vi "Lab Panel V4.87.vi"() -> ()   [LabVIEW 2013] (continued)
                n1786 = property on="JIG TEST" class="Clust (strict)"() -> ("DisabledEnum"=w3336:T16)  [unwired: 2 in, 2 out]
                n1787 = Equal?(x=w3336, y=2) -> (x = y?=w3335:bool)
                n1788 = Equal?(x=w3339, y=0) -> (x = y?=w3337:bool)
                n1789 = And(x=w3337, y=w3335) -> (x .and. y?=w3334:bool)
                n1790 = case shown="True" w3334 {
                  frame False {
                  }
                  frame True {
                    n1791 = local read "run lab01-1"() -> (w3350:bool)
                    n1792 = local read "run lab01-2"() -> (w3349:bool)
                    n1793 = local read "run lab02-1"() -> (w3348:bool)
                    n1794 = local read "run lab02-2"() -> (w3347:bool)
                    n1795 = local read "run lab03-1"() -> (w3346:bool)
                    n1796 = local read "run lab03-2"() -> (w3345:bool)
                    n1797 = local read "run lab04-1"() -> (w3344:bool)
                    n1798 = local read "run lab04-2"() -> (w3343:bool)
                    n1799 = local read "run lab05-1"() -> (w3342:bool)
                    n1800 = local read "run lab05-2"() -> (w3341:bool)
                    n1801 = local write "JIG LAB03-2"(w3345) -> ()
                    n1802 = local write "JIG LAB01-1"(w3350) -> ()
                    n1803 = local write "JIG LAB01-2"(w3349) -> ()
                    n1804 = local write "JIG LAB02-1"(w3348) -> ()
                    n1805 = local write "JIG LAB02-2"(w3347) -> ()
                    n1806 = local write "JIG LAB03-1"(w3346) -> ()
                    n1807 = local write "JIG LAB04-1"(w3344) -> ()
                    n1808 = local write "JIG LAB04-2"(w3343) -> ()
                    n1809 = local write "JIG LAB05-1"(w3342) -> ()
                    n1810 = local write "JIG LAB05-2"(w3341) -> ()
                  }
                }
              }
              frame #1 {
                # "jig off"
                n1811 = local read "jig cycle"() -> (w3357:dbl)
                n1812 = local read "on loops"() -> (w3356:dbl)
                n1813 = property on="JIG TEST" class="Clust (strict)"() -> ("DisabledEnum"=w3355:T16)  [unwired: 2 in, 2 out]
                n1814 = Equal?(x=w3355, y=2) -> (x = y?=w3353:bool)
                n1815 = Equal?(x=w3357, y=w3356) -> (x = y?=w3352:bool)
                n1816 = And(x=w3352, y=w3353) -> (x .and. y?=w3351:bool)
                n1817 = case shown="True" w3351 {
                  frame False {
                  }
                  frame True {
                    w3408 = FALSE
                    w3409 = TRUE
                    w3407 = 2
                    n1818 = local read "SELECT LAB05-2"() -> (w3398:T3)
                    n1819 = local read "SELECT LAB04-2"() -> (w3400:T3)
                    n1820 = local read "SELECT LAB04-1"() -> (w3401:T3)
                    n1821 = local read "SELECT LAB05-1"() -> (w3399:T3)
                    n1822 = local read "SELECT LAB03-2"() -> (w3402:T3)
                    n1823 = local read "SELECT LAB02-1"() -> (w3405:T3)
                    n1824 = local read "SELECT LAB03-1"() -> (w3403:T3)
                    n1825 = local read "SELECT LAB02-2"() -> (w3404:T3)
                    n1826 = local read "SELECT LAB01-2"() -> (w3406:T3)
                    n1827 = local read "run lab05-1"() -> (w3368:bool)
                    n1828 = local read "run lab05-2"() -> (w3367:bool)
                    n1829 = local read "SELECT LAB01-1"() -> (w3410:T3)
                    n1830 = local read "run lab04-2"() -> (w3369:bool)
                    n1831 = local read "run lab04-1"() -> (w3370:bool)
                    n1832 = local read "run lab01-1"() -> (w3386:bool)
                    n1833 = local read "run lab01-2"() -> (w3375:bool)
                    n1834 = local read "run lab03-2"() -> (w3371:bool)
                    n1835 = local read "run lab03-1"() -> (w3372:bool)
                    n1836 = local read "run lab02-1"() -> (w3374:bool)
                    n1837 = local read "run lab02-2"() -> (w3373:bool)
                    n1838 = Equal?(x=w3407, y=w3403) -> (x = y?=w3381:bool)
                    n1839 = Equal?(x=w3407, y=w3402) -> (x = y?=w3380:bool)
                    n1840 = Equal?(x=w3407, y=w3401) -> (x = y?=w3379:bool)
                    n1841 = Equal?(x=w3407, y=w3400) -> (x = y?=w3378:bool)
                    n1842 = Equal?(x=w3407, y=w3399) -> (x = y?=w3377:bool)
                    n1843 = Equal?(x=w3407, y=w3398) -> (x = y?=w3376:bool)
                    n1844 = Equal?(x=w3407, y=w3410) -> (x = y?=w3387:bool)
                    n1845 = Equal?(x=w3407, y=w3405) -> (x = y?=w3383:bool)
                    n1846 = Equal?(x=w3407, y=w3404) -> (x = y?=w3382:bool)
                    n1847 = Equal?(x=w3407, y=w3406) -> (x = y?=w3384:bool)
                    n1848 = And(x=w3378, y=w3369) -> (x .and. y?=w3360:bool)
                    n1849 = And(x=w3381, y=w3372) -> (x .and. y?=w3363:bool)
                    n1850 = And(x=w3379, y=w3370) -> (x .and. y?=w3361:bool)
                    n1851 = And(x=w3376, y=w3367) -> (x .and. y?=w3358:bool)
                    n1852 = And(x=w3382, y=w3373) -> (x .and. y?=w3364:bool)
                    n1853 = And(x=w3380, y=w3371) -> (x .and. y?=w3362:bool)
                    n1854 = And(x=w3377, y=w3368) -> (x .and. y?=w3359:bool)
                    n1855 = And(x=w3384, y=w3375) -> (x .and. y?=w3366:bool)
                    n1856 = And(x=w3387, y=w3386) -> (x .and. y?=w3385:bool)
                    n1857 = And(x=w3383, y=w3374) -> (x .and. y?=w3365:bool)
                    n1858 = Select(t=w3409, s=w3385, f=w3408) -> (s? t:f=w3388:bool)
                    n1859 = Select(t=w3409, s=w3366, f=w3408) -> (s? t:f=w3389:bool)
                    n1860 = Select(t=w3409, s=w3365, f=w3408) -> (s? t:f=w3390:bool)
                    n1861 = Select(t=w3409, s=w3364, f=w3408) -> (s? t:f=w3391:bool)
                    n1862 = Select(t=w3409, s=w3363, f=w3408) -> (s? t:f=w3392:bool)
                    n1863 = Select(t=w3409, s=w3362, f=w3408) -> (s? t:f=w3393:bool)
                    n1864 = Select(t=w3409, s=w3361, f=w3408) -> (s? t:f=w3394:bool)
                    n1865 = Select(t=w3409, s=w3360, f=w3408) -> (s? t:f=w3395:bool)
                    n1866 = Select(t=w3409, s=w3359, f=w3408) -> (s? t:f=w3396:bool)
                    n1867 = Select(t=w3409, s=w3358, f=w3408) -> (s? t:f=w3397:bool)
                    n1868 = local write "JIG LAB03-2"(w3393) -> ()
                    n1869 = local write "JIG LAB02-1"(w3390) -> ()
                    n1870 = local write "JIG LAB02-2"(w3391) -> ()
                    n1871 = local write "JIG LAB01-2"(w3389) -> ()
                    n1872 = local write "JIG LAB03-1"(w3392) -> ()
                    n1873 = local write "JIG LAB01-1"(w3388) -> ()
                    n1874 = local write "JIG LAB05-2"(w3397) -> ()
                    n1875 = local write "JIG LAB04-1"(w3394) -> ()
                    n1876 = local write "JIG LAB05-1"(w3396) -> ()
                    n1877 = local write "JIG LAB04-2"(w3395) -> ()
                  }
                }
              }
            }
          }
          frame #9 {
            # "enable  jig test output if no test busy"
            n1878 = property on="JIG TEST" class="Clust (strict)"() -> ("DisabledEnum"=w3413:T16)  [unwired: 2 in, 2 out]
            n1879 = Equal?(x=w3413, y=0) -> (x = y?=w3411:bool)
            n1880 = case shown="True" w3411 {
              frame False {
              }
              frame True {
                n1881 = local read "JIG TEST"() -> (w3424:T10)
                n1882 = Unbundle(w3424) -> ("LAB01-1"=w3423:bool, "LAB01-2"=w3422:bool, "LAB02-1"=w3421:bool, "LAB02-2"=w3420:bool, "LAB03-1"=w3419:bool, "LAB03-2"=w3418:bool, "LAB04-1"=w3417:bool, "LAB04-2"=w3416:bool, "LAB05-1"=w3415:bool, "LAB05-2"=w3414:bool)
                n1883 = local write "JIG LAB05-1"(w3415) -> ()
                n1884 = local write "JIG LAB05-2"(w3414) -> ()
                n1885 = local write "JIG LAB04-1"(w3417) -> ()
                n1886 = local write "JIG LAB04-2"(w3416) -> ()
                n1887 = local write "JIG LAB03-2"(w3418) -> ()
                n1888 = local write "JIG LAB01-1"(w3423) -> ()
                n1889 = local write "JIG LAB02-1"(w3421) -> ()
                n1890 = local write "JIG LAB03-1"(w3419) -> ()
                n1891 = local write "JIG LAB01-2"(w3422) -> ()
                n1892 = local write "JIG LAB02-2"(w3420) -> ()
              }
            }
          }
          frame #10 {
            # "drive digital output"
            n1893 = local read "O/I  LAB05-2"() -> (w3431:bool)
            n1894 = local read "O/I  LAB05-1"() -> (w3433:bool)
            n1895 = local read "JIG LAB05-2"() -> (w3430:bool)
            n1896 = local read "O/I  LAB04-2"() -> (w3435:bool)
            n1897 = local read "JIG LAB05-1"() -> (w3432:bool)
            n1898 = local read "JIG LAB04-2"() -> (w3434:bool)
            n1899 = local read "O/I  LAB03-1"() -> (w3440:bool)
            n1900 = local read "O/I  LAB04-1"() -> (w3436:bool)
            n1901 = local read "O/I  LAB02-1"() -> (w3444:bool)
            n1902 = local read "O/I  LAB02-2"() -> (w3442:bool)
            n1903 = local read "O/I  LAB03-2"() -> (w3438:bool)
            n1904 = local read "JIG LAB04-1"() -> (w3429:bool)
            n1905 = local read "JIG LAB03-2"() -> (w3437:bool)
            n1906 = local read "O/I  LAB01-2"() -> (w3446:bool)
            n1907 = local read "JIG LAB02-1"() -> (w3443:bool)
            n1908 = local read "JIG LAB02-2"() -> (w3441:bool)
            n1909 = local read "JIG LAB03-1"() -> (w3439:bool)
            n1910 = local read "O/I  LAB01-1"() -> (w3448:bool)
            n1911 = local read "JIG LAB01-2"() -> (w3445:bool)
            n1912 = local read "JIG LAB01-1"() -> (w3447:bool)
            n1913 = Build Array(w3435, w3434, w3433, w3432, w3431, w3430) -> (w3426:bool[])
            n1914 = Build Array(w3441, w3440, w3439, w3438, w3437, w3436, w3429) -> (w3427:bool[])
            n1915 = Build Array(w3448, w3447, w3446, w3445, w3444, w3443, w3442) -> (w3428:bool[])
            n1916 = local read "simulate"() -> (w3425:bool)
            n1917 = case shown="False" w3425 {
              tunnel: w3428 -> [w3451 _]
              tunnel: w3427 -> [w3450 _]
              tunnel: w3426 -> [w3449 _]
              frame False {
                n1918 = call "sub vi - Drive Relays All v6.vi"("Array #2"=w3449, "Array #1"=w3450, "Array #0"=w3451) -> ()  [unwired: 8 in, 1 out]
              }
              frame True {
              }
            }
          }
          frame #11 {
            # "get analog values"
            n1919 = local read "on loops"() -> (w3458:dbl)
            n1920 = local read "jig cycle"() -> (w3455:dbl)
            n1921 = Add(x=w3458, y=1) -> (x+y=w3456:dbl)
            n1922 = Equal?(x=w3455, y=1) -> (x = y?=w3452:bool)
            n1923 = Equal?(x=w3455, y=w3456) -> (x = y?=w3454:bool)
            n1924 = Or(x=w3452, y=w3454) -> (x .or. y?=w3453:bool)
            n1925 = global write "Global display 3.vi" "cycle O/F"(w3452) -> ()
            n1926 = case shown="True" w3453 {
              tunnel: w3452 -> [_ w3460]
              frame False {
              }
              frame True {
                n1927 = local read "simulate"() -> (w3463:bool)
                n1928 = case shown="True" w3463 {
                  tunnel: [w3472 errorcluster[] [] ("array ERROR")] -> w3471
                  tunnel: [w3479 0.3 ("Analog loop time")] -> w3470
                  tunnel: [w3478 dynamicdata[] [] ("array GRAPH")] -> w3469
                  tunnel: [w3477 w3480] -> w3468
                  tunnel: [w3476 w3480] -> w3467
                  tunnel: [w3475 w3480] -> w3466
                  tunnel: [w3474 w3480] -> w3465
                  tunnel: [w3473 w3480] -> w3464
                  tunnel: w3460 -> [_ w3486]
                  frame False {
                    n1929 = call "sub vi - Read Analog All v8.11.vi"() -> ("Analog loop time"=w3479:dbl, "array GRAPH"=w3478:dynamicdata[], "LAB01"=w3477:T26, "LAB02"=w3476:T27, "LAB03"=w3475:T28, "LAB04"=w3474:T29, "array ERROR"=w3472:errorcluster[], "LAB05"=w3473:T30)  [unwired: 8 in]
                  }
                  frame True {
                    n1930 = local read "ON amps"() -> (w3485:dbl)
                    n1931 = local read "OFF amps"() -> (w3484:dbl)
                    n1932 = local read "VOLTS"() -> (w3482:dbl)
                    n1933 = local read "PF"() -> (w3481:dbl)
                    n1934 = Select(t=w3485, s=w3486, f=w3484) -> (s? t:f=w3483:dbl)
                    n1935 = Bundle("OFF amps"=w3483, "VOLTS"=w3482, "PF"=w3481, "OFF amps"=w3483, "VOLTS"=w3482, "PF"=w3481) -> (w3480:T31)  [unwired: 1 in]
                  }
                }
                n1936 = local read "simulate"() -> (w3462:bool)
                n1937 = stacked-sequence {
                  tunnel: w3471 -> [w3494 _ _ _ _ _]
                  tunnel: w3470 -> [w3493 _ _ _ _ _]
                  tunnel: w3469 -> [w3490 _ _ _ _ _]
                  tunnel: w3468 -> [_ w3541 _ _ _ _]
                  tunnel: w3467 -> [_ _ w3548 _ _ _]
                  tunnel: w3466 -> [_ _ _ w3577 _ _]
                  tunnel: w3465 -> [_ _ _ _ w3604 _]
                  tunnel: w3464 -> [_ _ _ _ _ w3633]
                  tunnel: w3462 -> [_ w3519 w3547 w3575 w3603 w3631]
                  tunnel: T14 {"1  (A) cal"=1.0, "1 (V) cal"=1.0, "1 (PF) cal"=1.0, "1 (TL) cal"=1.0, "1 (TN) cal"=1.0, "2 (A) cal"=1.0, "2 (V) cal"=1.0, "2 (PF) cal"=1.0, "2 (TL) cal"=1.0, "2 (TN) cal"=1.0} ("CAL LAB01") -> [_ w3518 w3546 w3574 w3602 w3630]
                  frame #0 {
                    n1938 = local write "AI"(TRUE) -> ()
                    n1939 = global write "Global 1.vi" "RATE(Hz)"("RATE (Hz)") -> ()
                    n1940 = global write "Global 1.vi" "SAMPLES"("SAMPLES") -> ()
                    n1941 = Index Array(array=w3490, index=6) -> (element=→"LAB04-1 (GRAPH)":dynamicdata)
                    n1942 = Index Array(array=w3490, index=7) -> (element=→"LAB04-2 (GRAPH)":dynamicdata)
                    n1943 = Index Array(array=w3490, index=9) -> (element=→"LAB05-2 (GRAPH)":dynamicdata)
                    n1944 = Index Array(array=w3490, index=8) -> (element=→"LAB05-1 (GRAPH)":dynamicdata)
                    n1945 = Index Array(array=w3490, index=5) -> (element=→"LAB03-2 (GRAPH)":dynamicdata)
                    n1946 = Index Array(array=w3490, index=0) -> (element=→"LAB01-1 (GRAPH)":dynamicdata)
                    n1947 = Index Array(array=w3490, index=1) -> (element=→"LAB01-2 (GRAPH)":dynamicdata)
                    n1948 = Index Array(array=w3490, index=2) -> (element=→"LAB02-1 (GRAPH)":dynamicdata)
                    n1949 = Index Array(array=w3490, index=3) -> (element=→"LAB02-2 (GRAPH)":dynamicdata)
                    n1950 = Index Array(array=w3490, index=4) -> (element=→"LAB03-1 (GRAPH)":dynamicdata)
                    "AI loop time" <- w3493
                    "Analog Error Array" <- w3494
                  }
                  frame #1 {
                    n1951 = case shown="False" w3519 {
                      tunnel: [w3542 w3543] -> w3540
                      tunnel: w3518 -> [_ w3543]
                      frame False {
                        n1952 = local read "CAL LAB01"() -> (w3542:T14)
                      }
                      frame True {
                      }
                    }
                    n1953 = Unbundle By Name(w3541) -> ("OFF amps"=w3539:dbl, "VOLTS"=w3538:dbl, "PF"=w3537:dbl, "OFF amps"=w3536:dbl, "VOLTS"=w3535:dbl, "PF"=w3534:dbl)
                    n1954 = Unbundle By Name(w3540) -> ("1  (A) cal"=w3533:dbl, "1 (V) cal"=w3532:dbl, "1 (PF) cal"=w3531:dbl, "2 (A) cal"=w3530:dbl, "2 (V) cal"=w3529:dbl, "2 (PF) cal"=w3528:dbl)  [unwired: 4 out]
                    n1955 = Multiply(x=w3539, y=w3533) -> (x*y=w3526:dbl)
                    n1956 = Multiply(x=w3538, y=w3532) -> (x*y=w3525:dbl)
                    n1957 = Multiply(x=w3537, y=w3531) -> (x*y=w3524:dbl)
                    n1958 = Multiply(x=w3536, y=w3530) -> (x*y=w3522:dbl)
                    n1959 = Multiply(x=w3535, y=w3529) -> (x*y=w3521:dbl)
                    n1960 = Multiply(x=w3534, y=w3528) -> (x*y=w3520:dbl)
                    n1961 = local read "SIG LAB01-1"() -> (w3527:T2)
                    n1962 = local read "SIG LAB01-2"() -> (w3523:T2)
                    n1963 = Bundle By Name(cluster=w3527, "AMPS"=w3526, "VOLTS"=w3525, "PF"=w3524) -> (w3517:T2)
                    n1964 = Bundle By Name(cluster=w3523, "AMPS"=w3522, "VOLTS"=w3521, "PF"=w3520) -> (w3516:T2)
                    n1965 = global write "Global display 1.vi" "SIG LAB01-2"(w3516) -> ()
                    n1966 = global write "Global display 1.vi" "SIG LAB01-1"(w3517) -> ()
                    n1967 = local write "SIG LAB01-2"(w3516) -> ()
                    n1968 = local write "SIG LAB01-1"(w3517) -> ()
                  }
                  frame #2 {
                    n1969 = Unbundle By Name(w3548) -> ("OFF amps"=w3568:dbl, "VOLTS"=w3567:dbl, "PF"=w3566:dbl, "OFF amps"=w3565:dbl, "VOLTS"=w3564:dbl, "PF"=w3563:dbl)
                    n1970 = case shown="True" w3547 {
                      tunnel: [w3570 w3571] -> w3569
                      tunnel: w3546 -> [_ w3571]
                      frame False {
                        n1971 = local read "CAL LAB02"() -> (w3570:T15)
                      }
                      frame True {
                      }
                    }
                    n1972 = Unbundle By Name(w3569) -> ("1  (A) cal"=w3562:dbl, "1 (V) cal"=w3561:dbl, "1 (PF) cal"=w3560:dbl, "2 (A) cal"=w3559:dbl, "2 (V) cal"=w3558:dbl, "2 (PF) cal"=w3557:dbl)  [unwired: 4 out]
                    n1973 = Multiply(x=w3568, y=w3562) -> (x*y=w3555:dbl)
                    n1974 = Multiply(x=w3567, y=w3561) -> (x*y=w3554:dbl)
                    n1975 = Multiply(x=w3566, y=w3560) -> (x*y=w3553:dbl)
                    n1976 = Multiply(x=w3565, y=w3559) -> (x*y=w3551:dbl)
                    n1977 = Multiply(x=w3564, y=w3558) -> (x*y=w3550:dbl)
                    n1978 = Multiply(x=w3563, y=w3557) -> (x*y=w3549:dbl)
                    n1979 = local read "SIG LAB02-1"() -> (w3556:T2)
                    n1980 = local read "SIG LAB02-2"() -> (w3552:T2)
                    n1981 = Bundle By Name(cluster=w3556, "AMPS"=w3555, "VOLTS"=w3554, "PF"=w3553) -> (w3545:T2)
                    n1982 = Bundle By Name(cluster=w3552, "AMPS"=w3551, "VOLTS"=w3550, "PF"=w3549) -> (w3544:T2)
                    n1983 = global write "Global display 1.vi" "SIG LAB02-1"(w3545) -> ()
                    n1984 = local write "SIG LAB02-2"(w3544) -> ()
                    n1985 = global write "Global display 1.vi" "SIG LAB02-2"(w3544) -> ()
                    n1986 = local write "SIG LAB02-1"(w3545) -> ()
                  }
                  frame #3 {
                    n1987 = Unbundle By Name(w3577) -> ("OFF amps"=w3596:dbl, "VOLTS"=w3595:dbl, "PF"=w3594:dbl, "OFF amps"=w3593:dbl, "VOLTS"=w3592:dbl, "PF"=w3591:dbl)
                    n1988 = case shown="True" w3575 {
                      tunnel: [w3598 w3599] -> w3597
                      tunnel: w3574 -> [_ w3599]
                      frame False {
                        n1989 = local read "CAL LAB03"() -> (w3598:T14)
                      }
                      frame True {
                      }
                    }
                    n1990 = Unbundle By Name(w3597) -> ("1  (A) cal"=w3590:dbl, "1 (V) cal"=w3589:dbl, "1 (PF) cal"=w3588:dbl, "2 (A) cal"=w3587:dbl, "2 (V) cal"=w3586:dbl, "2 (PF) cal"=w3585:dbl)  [unwired: 4 out]
                    n1991 = Multiply(x=w3596, y=w3590) -> (x*y=w3583:dbl)
                    n1992 = Multiply(x=w3595, y=w3589) -> (x*y=w3576:dbl)
                    n1993 = Multiply(x=w3594, y=w3588) -> (x*y=w3582:dbl)
                    n1994 = Multiply(x=w3593, y=w3587) -> (x*y=w3580:dbl)
                    n1995 = Multiply(x=w3592, y=w3586) -> (x*y=w3579:dbl)
                    n1996 = Multiply(x=w3591, y=w3585) -> (x*y=w3578:dbl)
                    n1997 = local read "SIG LAB03-1"() -> (w3584:T2)
                    n1998 = local read "SIG LAB03-2"() -> (w3581:T2)
                    n1999 = Bundle By Name(cluster=w3584, "AMPS"=w3583, "VOLTS"=w3576, "PF"=w3582) -> (w3573:T2)
                    n2000 = Bundle By Name(cluster=w3581, "AMPS"=w3580, "VOLTS"=w3579, "PF"=w3578) -> (w3572:T2)
                    n2001 = global write "Global display 1.vi" "SIG LAB03-1"(w3573) -> ()
                    n2002 = global write "Global display 1.vi" "SIG LAB03-2"(w3572) -> ()
                    n2003 = local write "SIG LAB03-2"(w3572) -> ()
                    n2004 = local write "SIG LAB03-1"(w3573) -> ()
                  }
                  frame #4 {
                    n2005 = Unbundle By Name(w3604) -> ("OFF amps"=w3624:dbl, "VOLTS"=w3623:dbl, "PF"=w3622:dbl, "OFF amps"=w3621:dbl, "VOLTS"=w3620:dbl, "PF"=w3619:dbl)
                    n2006 = case shown="False" w3603 {
                      tunnel: [w3626 w3627] -> w3625
                      tunnel: w3602 -> [_ w3627]
                      frame False {
                        n2007 = local read "CAL LAB04"() -> (w3626:T14)
                      }
                      frame True {
                      }
                    }
                    n2008 = Unbundle By Name(w3625) -> ("1  (A) cal"=w3618:dbl, "1 (V) cal"=w3617:dbl, "1 (PF) cal"=w3616:dbl, "2 (A) cal"=w3615:dbl, "2 (V) cal"=w3614:dbl, "2 (PF) cal"=w3613:dbl)  [unwired: 4 out]
                    n2009 = Multiply(x=w3624, y=w3618) -> (x*y=w3611:dbl)
                    n2010 = Multiply(x=w3623, y=w3617) -> (x*y=w3610:dbl)
                    n2011 = Multiply(x=w3622, y=w3616) -> (x*y=w3609:dbl)
                    n2012 = Multiply(x=w3621, y=w3615) -> (x*y=w3607:dbl)
                    n2013 = Multiply(x=w3620, y=w3614) -> (x*y=w3606:dbl)
                    n2014 = Multiply(x=w3619, y=w3613) -> (x*y=w3605:dbl)
                    n2015 = local read "SIG LAB04-1"() -> (w3612:T2)
                    n2016 = local read "SIG LAB04-2"() -> (w3608:T2)
                    n2017 = Bundle By Name(cluster=w3612, "AMPS"=w3611, "VOLTS"=w3610, "PF"=w3609) -> (w3601:T2)
                    n2018 = Bundle By Name(cluster=w3608, "AMPS"=w3607, "VOLTS"=w3606, "PF"=w3605) -> (w3600:T2)
                    n2019 = global write "Global display 1.vi" "SIG LAB04-2"(w3600) -> ()
                    n2020 = global write "Global display 1.vi" "SIG LAB04-1"(w3601) -> ()
                    n2021 = local write "SIG LAB04-2"(w3600) -> ()
                    n2022 = local write "SIG LAB04-1"(w3601) -> ()
                  }
                  frame #5 {
                    n2023 = Unbundle By Name(w3633) -> ("OFF amps"=w3652:dbl, "VOLTS"=w3632:dbl, "PF"=w3651:dbl, "OFF amps"=w3650:dbl, "VOLTS"=w3649:dbl, "PF"=w3648:dbl)
                    n2024 = case shown="False" w3631 {
                      tunnel: [w3654 w3655] -> w3653
                      tunnel: w3630 -> [_ w3655]
                      frame False {
                        n2025 = local read "CAL LAB05"() -> (w3654:T14)
                      }
                      frame True {
                      }
                    }
                    n2026 = Unbundle By Name(w3653) -> ("1  (A) cal"=w3647:dbl, "1 (V) cal"=w3646:dbl, "1 (PF) cal"=w3645:dbl, "2 (A) cal"=w3644:dbl, "2 (V) cal"=w3643:dbl, "2 (PF) cal"=w3642:dbl)  [unwired: 4 out]
                    n2027 = Multiply(x=w3652, y=w3647) -> (x*y=w3640:dbl)
                    n2028 = Multiply(x=w3632, y=w3646) -> (x*y=w3639:dbl)
                    n2029 = Multiply(x=w3651, y=w3645) -> (x*y=w3638:dbl)
                    n2030 = Multiply(x=w3650, y=w3644) -> (x*y=w3636:dbl)
                    n2031 = Multiply(x=w3649, y=w3643) -> (x*y=w3635:dbl)
                    n2032 = Multiply(x=w3648, y=w3642) -> (x*y=w3634:dbl)
                    n2033 = local read "SIG LAB05-1"() -> (w3641:T2)
                    n2034 = local read "SIG LAB05-2"() -> (w3637:T2)
                    n2035 = Bundle By Name(cluster=w3641, "AMPS"=w3640, "VOLTS"=w3639, "PF"=w3638) -> (w3629:T2)
                    n2036 = Bundle By Name(cluster=w3637, "AMPS"=w3636, "VOLTS"=w3635, "PF"=w3634) -> (w3628:T2)
                    n2037 = global write "Global display 1.vi" "SIG LAB05-1"(w3629) -> ()
                    n2038 = global write "Global display 1.vi" "SIG LAB05-2"(w3628) -> ()
                    n2039 = local write "SIG LAB05-2"(w3628) -> ()
                    n2040 = local write "SIG LAB05-1"(w3629) -> ()
                  }
                }
              }
            }
          }
          frame #12 {
            # "save test data to file"
            n2041 = Get Date/Time In Seconds() -> (seconds since 1Jan1904=w3656:timestamp)
            "File Time Stamp" <- w3656
            n2042 = local read "on loops"() -> (w3675:dbl)
            n2043 = local read "jig cycle"() -> (w3672:dbl)
            n2044 = Format Date/Time String(time format string (%c)="%H:%M%:%S", seconds (now)=w3656) -> (date/time string=w3660:string)  [unwired: 1 in]
            n2045 = Add(x=w3675, y=2) -> (x+y=w3673:dbl)
            n2046 = Build Array(w3660) -> (w3659:string[])
            n2047 = Equal?(x=w3672, y=1) -> (x = y?=w3658:bool)
            n2048 = Equal?(x=w3672, y=w3673) -> (x = y?=w3657:bool)
            n2049 = stacked-sequence {
              tunnel: w3671 -> [w3681 _ _ _ _ _ _ _ _ _]
              tunnel: w3670 -> [_ w3757 _ _ _ _ _ _ _ _]
              tunnel: w3669 -> [_ _ w3837 _ _ _ _ _ _ _]
              tunnel: w3668 -> [_ _ _ w3917 _ _ _ _ _ _]
              tunnel: w3667 -> [_ _ _ _ w3997 _ _ _ _ _]
              tunnel: w3666 -> [_ _ _ _ _ w4077 _ _ _ _]
              tunnel: w3665 -> [_ _ _ _ _ _ w4157 _ _ _]
              tunnel: w3664 -> [_ _ _ _ _ _ _ w4237 _ _]
              tunnel: w3663 -> [_ _ _ _ _ _ _ _ w4317 _]
              tunnel: w3662 -> [_ _ _ _ _ _ _ _ _ w4397]
              tunnel: w3659 -> [w3680 w3761 w3841 w3921 w4001 w4081 w4161 w4241 w4321 w4401]
              tunnel: w3658 -> [w3679 w3760 w3840 w3920 w4000 w4080 w4160 w4240 w4320 w4400]
              tunnel: w3657 -> [w3678 w3759 w3839 w3919 w3999 w4079 w4159 w4239 w4319 w4399]
              tunnel: w3656 -> [w3677 w3758 w3838 w3918 w3998 w4078 w4158 w4238 w4318 w4398]
              frame #0 {
                n2050 = case shown="True" w3681 {
                  tunnel: w3680 -> [_ w3686]
                  tunnel: w3679 -> [_ w3685]
                  tunnel: w3678 -> [_ w3683]
                  tunnel: w3677 -> [_ w3682]
                  frame False {
                  }
                  frame True {
                    n2051 = local read "DISP LAB01-1"() -> (w3687:T4)
                    n2052 = local read "SIG LAB01-1"() -> (w3688:T2)
                    n2053 = local read "ON L01-1"() -> (w3684:cluster{"amps":dbl, "volts":dbl, "pf":dbl})
                    n2054 = Unbundle(w3688) -> ("AMPS"=w3694:dbl, "VOLTS"=w3692:dbl, "PF"=w3691:dbl, "Tmp Live"=w3690:dbl, "Tmp Neut"=w3693:dbl)
                    n2055 = Unbundle(w3687) -> ("CYCLE"=w3689:dbl)  [unwired: 2 out]
                    n2056 = stacked-sequence {
                      tunnel: w3694 -> [w3698 w3717]
                      tunnel: w3693 -> [_ w3716]
                      tunnel: w3692 -> [w3697 w3715]
                      tunnel: w3691 -> [w3696 w3714]
                      tunnel: w3690 -> [_ w3713]
                      tunnel: w3689 -> [_ w3712]
                      tunnel: w3686 -> [_ w3711]
                      tunnel: w3685 -> [w3699 _]
                      tunnel: w3684 -> [w3695 w3709]
                      tunnel: w3683 -> [_ w3710]
                      tunnel: w3682 -> [_ w3705]
                      frame #0 {
                        n2057 = case shown="True" w3699 {
                          tunnel: w3698 -> [_ w3704]
                          tunnel: w3697 -> [_ w3703]
                          tunnel: w3696 -> [_ w3702]
                          tunnel: w3695 -> [_ w3700]
                          frame False {
                          }
                          frame True {
                            n2058 = Bundle(cluster=w3700, "amps"=w3704, "volts"=w3703, "pf"=w3702) -> (w3701:cluster{"amps":dbl, "volts":dbl, "pf":dbl})
                            n2059 = local write "ON L01-1"(w3701) -> ()
                          }
                        }
                      }
                      frame #1 {
                        n2060 = Unbundle(w3709) -> ("amps"=w3708:dbl, "volts"=w3707:dbl, "pf"=w3706:dbl)
                        n2061 = case shown="True" w3710 {
                          tunnel: w3717 -> [_ w3718]
                          tunnel: w3716 -> [_ w3756]
                          tunnel: w3715 -> [_ _]
                          tunnel: w3714 -> [_ _]
                          tunnel: w3713 -> [_ w3755]
                          tunnel: w3712 -> [_ w3754]
                          tunnel: w3711 -> [_ w3722]
                          tunnel: w3708 -> [_ w3719]
                          tunnel: w3707 -> [_ w3751]
                          tunnel: w3706 -> [_ w3750]
                          tunnel: w3705 -> [_ w3720]
                          frame False {
                          }
                          frame True {
                            n2062 = local read "TDMS LAB01-1"() -> (w3753:refnum<k34>)
                            n2063 = Build Array(w3751) -> (w3747:dbl[])
                            n2064 = Build Array(w3750) -> (w3746:dbl[])
                            n2065 = Build Array(w3755) -> (w3745:dbl[])
                            n2066 = Build Array(w3756) -> (w3744:dbl[])
                            n2067 = Build Array(w3719) -> (w3749:dbl[])
                            n2068 = Build Array(w3718) -> (w3748:dbl[])
                            n2069 = Build Array(w3754) -> (w3743:dbl[])
                            n2070 = Build Array("AMPS ON", "AMPS OFF", "VOLTS", "PF", "TEMP Live", "TEMP Neut", "CYCLE") -> (w3727:string[])
                            n2071 = Bundle By Name("Y"=w3749, "t0"=w3720) -> (w3742:waveform(dbl))  [unwired: 1 in]
                            n2072 = Bundle By Name("Y"=w3748, "t0"=w3720) -> (w3741:waveform(dbl))  [unwired: 1 in]
                            n2073 = Bundle By Name("Y"=w3747, "t0"=w3720) -> (w3740:waveform(dbl))  [unwired: 1 in]
                            n2074 = Bundle By Name("Y"=w3746, "t0"=w3720) -> (w3739:waveform(dbl))  [unwired: 1 in]
                            n2075 = Bundle By Name("Y"=w3745, "t0"=w3720) -> (w3738:waveform(dbl))  [unwired: 1 in]
                            n2076 = Bundle By Name("Y"=w3744, "t0"=w3720) -> (w3737:waveform(dbl))  [unwired: 1 in]
                            n2077 = Bundle By Name("Y"=w3743, "t0"=w3720) -> (w3736:waveform(dbl))  [unwired: 1 in]
                            n2078 = Build Array(w3742, w3741, w3740, w3739, w3738, w3737, w3736) -> (w3735:waveform(dbl)[])
                            n2079 = TDMS Write(0:w3753, 5:"TEST VALUES", 7:w3727, 9:w3735) -> (4:w3726:refnum<k34>, 6:w3725:string, 15:w3724:errorcluster)  [unwired: 2 in, 1 out]
                            n2080 = TDMS Write(0:w3726, 5:w3725, 7:"TIME", 9:w3722, 11:w3724) -> (15:w3721:errorcluster)  [unwired: 1 in, 3 out]
                            n2081 = local write "data file error"(w3721) -> ()
                          }
                        }
                      }
                    }
                  }
                }
              }
              frame #1 {
                n2082 = case shown="True" w3757 {
                  tunnel: w3761 -> [_ w3766]
                  tunnel: w3760 -> [_ w3765]
                  tunnel: w3759 -> [_ w3763]
                  tunnel: w3758 -> [_ w3762]
                  frame False {
                  }
                  frame True {
                    n2083 = local read "DISP LAB01-2"() -> (w3767:T4)
                    n2084 = local read "SIG LAB01-2"() -> (w3768:T2)
                    n2085 = local read "ON L01-2"() -> (w3764:cluster{"amps":dbl, "volts":dbl, "pf":dbl})
                    n2086 = Unbundle(w3768) -> ("AMPS"=w3774:dbl, "VOLTS"=w3772:dbl, "PF"=w3771:dbl, "Tmp Live"=w3770:dbl, "Tmp Neut"=w3773:dbl)
                    n2087 = Unbundle(w3767) -> ("CYCLE"=w3769:dbl)  [unwired: 2 out]
                    n2088 = stacked-sequence {
                      tunnel: w3774 -> [w3778 w3797]
                      tunnel: w3773 -> [_ w3796]
                      tunnel: w3772 -> [w3777 w3795]
                      tunnel: w3771 -> [w3776 w3794]
                      tunnel: w3770 -> [_ w3793]
                      tunnel: w3769 -> [_ w3792]
                      tunnel: w3766 -> [_ w3791]
                      tunnel: w3765 -> [w3779 _]
                      tunnel: w3764 -> [w3775 w3789]
                      tunnel: w3763 -> [_ w3790]
                      tunnel: w3762 -> [_ w3785]
                      frame #0 {
                        n2089 = case shown="True" w3779 {
                          tunnel: w3778 -> [_ w3784]
                          tunnel: w3777 -> [_ w3783]
                          tunnel: w3776 -> [_ w3782]
                          tunnel: w3775 -> [_ w3780]
                          frame False {
                          }
                          frame True {
                            n2090 = Bundle(cluster=w3780, "amps"=w3784, "volts"=w3783, "pf"=w3782) -> (w3781:cluster{"amps":dbl, "volts":dbl, "pf":dbl})
                            n2091 = local write "ON L01-2"(w3781) -> ()
                          }
                        }
                      }
                      frame #1 {
                        n2092 = Unbundle(w3789) -> ("amps"=w3788:dbl, "volts"=w3787:dbl, "pf"=w3786:dbl)
                        n2093 = case shown="True" w3790 {
                          tunnel: w3797 -> [_ w3829]
                          tunnel: w3796 -> [_ w3836]
                          tunnel: w3795 -> [_ _]
                          tunnel: w3794 -> [_ _]
                          tunnel: w3793 -> [_ w3835]
                          tunnel: w3792 -> [_ w3834]
                          tunnel: w3791 -> [_ w3799]
                          tunnel: w3788 -> [_ w3831]
                          tunnel: w3787 -> [_ w3830]
                          tunnel: w3786 -> [_ w3828]
                          tunnel: w3785 -> [_ w3820]
                          frame False {
                          }
                          frame True {
                            n2094 = local read "TDMS LAB01-2"() -> (w3833:refnum<k34>)
                            n2095 = Build Array(w3830) -> (w3825:dbl[])
                            n2096 = Build Array(w3828) -> (w3824:dbl[])
                            n2097 = Build Array(w3835) -> (w3823:dbl[])
                            n2098 = Build Array(w3836) -> (w3822:dbl[])
                            n2099 = Build Array(w3831) -> (w3827:dbl[])
                            n2100 = Build Array(w3829) -> (w3826:dbl[])
                            n2101 = Build Array(w3834) -> (w3821:dbl[])
                            n2102 = Build Array("AMPS ON", "AMPS OFF", "VOLTS", "PF", "TEMP Live", "TEMP Neut", "CYCLE") -> (w3804:string[])
                            n2103 = Bundle By Name("Y"=w3827, "t0"=w3820) -> (w3819:waveform(dbl))  [unwired: 1 in]
                            n2104 = Bundle By Name("Y"=w3826, "t0"=w3820) -> (w3818:waveform(dbl))  [unwired: 1 in]
                            n2105 = Bundle By Name("Y"=w3825, "t0"=w3820) -> (w3817:waveform(dbl))  [unwired: 1 in]
                            n2106 = Bundle By Name("Y"=w3824, "t0"=w3820) -> (w3816:waveform(dbl))  [unwired: 1 in]
                            n2107 = Bundle By Name("Y"=w3823, "t0"=w3820) -> (w3815:waveform(dbl))  [unwired: 1 in]
                            n2108 = Bundle By Name("Y"=w3822, "t0"=w3820) -> (w3814:waveform(dbl))  [unwired: 1 in]
                            n2109 = Bundle By Name("Y"=w3821, "t0"=w3820) -> (w3813:waveform(dbl))  [unwired: 1 in]
                            n2110 = Build Array(w3819, w3818, w3817, w3816, w3815, w3814, w3813) -> (w3812:waveform(dbl)[])
                            n2111 = TDMS Write(0:w3833, 5:"TEST VALUES", 7:w3804, 9:w3812) -> (4:w3803:refnum<k34>, 6:w3802:string, 15:w3801:errorcluster)  [unwired: 2 in, 1 out]
                            n2112 = TDMS Write(0:w3803, 5:w3802, 7:"TIME", 9:w3799, 11:w3801) -> (15:w3798:errorcluster)  [unwired: 1 in, 3 out]
                            n2113 = local write "data file error"(w3798) -> ()
                          }
                        }
                      }
                    }
                  }
                }
              }
              frame #2 {
                n2114 = case shown="True" w3837 {
                  tunnel: w3841 -> [_ w3846]
                  tunnel: w3840 -> [_ w3845]
                  tunnel: w3839 -> [_ w3843]
                  tunnel: w3838 -> [_ w3842]
                  frame False {
                  }
                  frame True {
                    n2115 = local read "DISP LAB02-1"() -> (w3847:T4)
                    n2116 = local read "SIG LAB02-1"() -> (w3848:T2)
                    n2117 = local read "ON L02-1"() -> (w3844:cluster{"amps":dbl, "volts":dbl, "pf":dbl})
                    n2118 = Unbundle(w3848) -> ("AMPS"=w3854:dbl, "VOLTS"=w3852:dbl, "PF"=w3851:dbl, "Tmp Live"=w3850:dbl, "Tmp Neut"=w3853:dbl)
                    n2119 = Unbundle(w3847) -> ("CYCLE"=w3849:dbl)  [unwired: 2 out]
                    n2120 = stacked-sequence {
                      tunnel: w3854 -> [w3858 w3877]
                      tunnel: w3853 -> [_ w3876]
                      tunnel: w3852 -> [w3857 w3875]
                      tunnel: w3851 -> [w3856 w3874]
                      tunnel: w3850 -> [_ w3873]
                      tunnel: w3849 -> [_ w3872]
                      tunnel: w3846 -> [_ w3871]
                      tunnel: w3845 -> [w3859 _]
                      tunnel: w3844 -> [w3855 w3869]
                      tunnel: w3843 -> [_ w3870]
                      tunnel: w3842 -> [_ w3865]
                      frame #0 {
                        n2121 = case shown="True" w3859 {
                          tunnel: w3858 -> [_ w3864]
                          tunnel: w3857 -> [_ w3863]
                          tunnel: w3856 -> [_ w3862]
                          tunnel: w3855 -> [_ w3860]
                          frame False {
                          }
                          frame True {
                            n2122 = Bundle(cluster=w3860, "amps"=w3864, "volts"=w3863, "pf"=w3862) -> (w3861:cluster{"amps":dbl, "volts":dbl, "pf":dbl})
                            n2123 = local write "ON L02-1"(w3861) -> ()
                          }
                        }
                      }
                      frame #1 {
                        n2124 = Unbundle(w3869) -> ("amps"=w3868:dbl, "volts"=w3867:dbl, "pf"=w3866:dbl)
                        n2125 = case shown="True" w3870 {
                          tunnel: w3877 -> [_ w3909]
                          tunnel: w3876 -> [_ w3916]
                          tunnel: w3875 -> [_ _]
                          tunnel: w3874 -> [_ _]
                          tunnel: w3873 -> [_ w3915]
                          tunnel: w3872 -> [_ w3914]
                          tunnel: w3871 -> [_ w3879]
                          tunnel: w3868 -> [_ w3911]
                          tunnel: w3867 -> [_ w3910]
                          tunnel: w3866 -> [_ w3908]
                          tunnel: w3865 -> [_ w3900]
                          frame False {
                          }
                          frame True {
                            n2126 = local read "TDMS LAB02-1"() -> (w3913:refnum<k34>)
                            n2127 = Build Array(w3910) -> (w3905:dbl[])
                            n2128 = Build Array(w3908) -> (w3904:dbl[])
                            n2129 = Build Array(w3915) -> (w3903:dbl[])
                            n2130 = Build Array(w3916) -> (w3902:dbl[])
                            n2131 = Build Array(w3911) -> (w3907:dbl[])
                            n2132 = Build Array(w3909) -> (w3906:dbl[])
                            n2133 = Build Array(w3914) -> (w3901:dbl[])
                            n2134 = Build Array("AMPS ON", "AMPS OFF", "VOLTS", "PF", "TEMP Live", "TEMP Neut", "CYCLE") -> (w3884:string[])
                            n2135 = Bundle By Name("Y"=w3907, "t0"=w3900) -> (w3899:waveform(dbl))  [unwired: 1 in]
                            n2136 = Bundle By Name("Y"=w3906, "t0"=w3900) -> (w3898:waveform(dbl))  [unwired: 1 in]
                            n2137 = Bundle By Name("Y"=w3905, "t0"=w3900) -> (w3897:waveform(dbl))  [unwired: 1 in]
                            n2138 = Bundle By Name("Y"=w3904, "t0"=w3900) -> (w3896:waveform(dbl))  [unwired: 1 in]
                            n2139 = Bundle By Name("Y"=w3903, "t0"=w3900) -> (w3895:waveform(dbl))  [unwired: 1 in]
                            n2140 = Bundle By Name("Y"=w3902, "t0"=w3900) -> (w3894:waveform(dbl))  [unwired: 1 in]
                            n2141 = Bundle By Name("Y"=w3901, "t0"=w3900) -> (w3893:waveform(dbl))  [unwired: 1 in]
                            n2142 = Build Array(w3899, w3898, w3897, w3896, w3895, w3894, w3893) -> (w3892:waveform(dbl)[])
                            n2143 = TDMS Write(0:w3913, 5:"TEST VALUES", 7:w3884, 9:w3892) -> (4:w3883:refnum<k34>, 6:w3882:string, 15:w3881:errorcluster)  [unwired: 2 in, 1 out]
                            n2144 = TDMS Write(0:w3883, 5:w3882, 7:"TIME", 9:w3879, 11:w3881) -> (15:w3878:errorcluster)  [unwired: 1 in, 3 out]
                            n2145 = local write "data file error"(w3878) -> ()
                          }
                        }
                      }
                    }
                  }
                }
              }
              frame #3 {
                n2146 = case shown="True" w3917 {
                  tunnel: w3921 -> [_ w3926]
                  tunnel: w3920 -> [_ w3925]
                  tunnel: w3919 -> [_ w3923]
                  tunnel: w3918 -> [_ w3922]
                  frame False {
                  }
                  frame True {
                    n2147 = local read "DISP LAB02-2"() -> (w3927:T4)
                    n2148 = local read "SIG LAB02-2"() -> (w3928:T2)
                    n2149 = local read "ON L02-2"() -> (w3924:cluster{"amps":dbl, "volts":dbl, "pf":dbl})
                    n2150 = Unbundle(w3928) -> ("AMPS"=w3934:dbl, "VOLTS"=w3932:dbl, "PF"=w3931:dbl, "Tmp Live"=w3930:dbl, "Tmp Neut"=w3933:dbl)
                    n2151 = Unbundle(w3927) -> ("CYCLE"=w3929:dbl)  [unwired: 2 out]
                    n2152 = stacked-sequence {
                      tunnel: w3934 -> [w3938 w3957]
                      tunnel: w3933 -> [_ w3956]
                      tunnel: w3932 -> [w3937 w3955]
                      tunnel: w3931 -> [w3936 w3954]
                      tunnel: w3930 -> [_ w3953]
                      tunnel: w3929 -> [_ w3952]
                      tunnel: w3926 -> [_ w3951]
                      tunnel: w3925 -> [w3939 _]
                      tunnel: w3924 -> [w3935 w3949]
                      tunnel: w3923 -> [_ w3950]
                      tunnel: w3922 -> [_ w3945]
                      frame #0 {
                        n2153 = case shown="True" w3939 {
                          tunnel: w3938 -> [_ w3944]
                          tunnel: w3937 -> [_ w3943]
                          tunnel: w3936 -> [_ w3942]
                          tunnel: w3935 -> [_ w3940]
                          frame False {
                          }
                          frame True {
                            n2154 = Bundle(cluster=w3940, "amps"=w3944, "volts"=w3943, "pf"=w3942) -> (w3941:cluster{"amps":dbl, "volts":dbl, "pf":dbl})
                            n2155 = local write "ON L02-2"(w3941) -> ()
                          }
                        }
                      }
                      frame #1 {
                        n2156 = Unbundle(w3949) -> ("amps"=w3948:dbl, "volts"=w3947:dbl, "pf"=w3946:dbl)
                        n2157 = case shown="True" w3950 {
                          tunnel: w3957 -> [_ w3989]
                          tunnel: w3956 -> [_ w3996]
                          tunnel: w3955 -> [_ _]
                          tunnel: w3954 -> [_ _]
                          tunnel: w3953 -> [_ w3995]
                          tunnel: w3952 -> [_ w3994]
                          tunnel: w3951 -> [_ w3959]
                          tunnel: w3948 -> [_ w3991]
                          tunnel: w3947 -> [_ w3990]
                          tunnel: w3946 -> [_ w3988]
                          tunnel: w3945 -> [_ w3980]
                          frame False {
                          }
                          frame True {
                            n2158 = local read "TDMS LAB02-2"() -> (w3993:refnum<k34>)
                            n2159 = Build Array(w3990) -> (w3985:dbl[])
                            n2160 = Build Array(w3988) -> (w3984:dbl[])
                            n2161 = Build Array(w3995) -> (w3983:dbl[])
                            n2162 = Build Array(w3996) -> (w3982:dbl[])
                            n2163 = Build Array(w3991) -> (w3987:dbl[])
                            n2164 = Build Array(w3989) -> (w3986:dbl[])
                            n2165 = Build Array(w3994) -> (w3981:dbl[])
                            n2166 = Build Array("AMPS ON", "AMPS OFF", "VOLTS", "PF", "TEMP Live", "TEMP Neut", "CYCLE") -> (w3964:string[])
                            n2167 = Bundle By Name("Y"=w3987, "t0"=w3980) -> (w3979:waveform(dbl))  [unwired: 1 in]
                            n2168 = Bundle By Name("Y"=w3986, "t0"=w3980) -> (w3978:waveform(dbl))  [unwired: 1 in]
                            n2169 = Bundle By Name("Y"=w3985, "t0"=w3980) -> (w3977:waveform(dbl))  [unwired: 1 in]
                            n2170 = Bundle By Name("Y"=w3984, "t0"=w3980) -> (w3976:waveform(dbl))  [unwired: 1 in]
                            n2171 = Bundle By Name("Y"=w3983, "t0"=w3980) -> (w3975:waveform(dbl))  [unwired: 1 in]
                            n2172 = Bundle By Name("Y"=w3982, "t0"=w3980) -> (w3974:waveform(dbl))  [unwired: 1 in]
                            n2173 = Bundle By Name("Y"=w3981, "t0"=w3980) -> (w3973:waveform(dbl))  [unwired: 1 in]
                            n2174 = Build Array(w3979, w3978, w3977, w3976, w3975, w3974, w3973) -> (w3972:waveform(dbl)[])
                            n2175 = TDMS Write(0:w3993, 5:"TEST VALUES", 7:w3964, 9:w3972) -> (4:w3963:refnum<k34>, 6:w3962:string, 15:w3961:errorcluster)  [unwired: 2 in, 1 out]
                            n2176 = TDMS Write(0:w3963, 5:w3962, 7:"TIME", 9:w3959, 11:w3961) -> (15:w3958:errorcluster)  [unwired: 1 in, 3 out]
                            n2177 = local write "data file error"(w3958) -> ()
                          }
                        }
                      }
                    }
                  }
                }
              }
              frame #4 {
                n2178 = case shown="True" w3997 {
                  tunnel: w4001 -> [_ w4006]
                  tunnel: w4000 -> [_ w4005]
                  tunnel: w3999 -> [_ w4003]
                  tunnel: w3998 -> [_ w4002]
                  frame False {
                  }
                  frame True {
                    n2179 = local read "DISP LAB03-1"() -> (w4007:T4)
                    n2180 = local read "SIG LAB03-1"() -> (w4008:T2)
                    n2181 = local read "ON L03-1"() -> (w4004:cluster{"amps":dbl, "volts":dbl, "pf":dbl})
                    n2182 = Unbundle(w4008) -> ("AMPS"=w4014:dbl, "VOLTS"=w4012:dbl, "PF"=w4011:dbl, "Tmp Live"=w4010:dbl, "Tmp Neut"=w4013:dbl)
                    n2183 = Unbundle(w4007) -> ("CYCLE"=w4009:dbl)  [unwired: 2 out]
                    n2184 = stacked-sequence {
                      tunnel: w4014 -> [w4018 w4037]
                      tunnel: w4013 -> [_ w4036]
                      tunnel: w4012 -> [w4017 w4035]
                      tunnel: w4011 -> [w4016 w4034]
                      tunnel: w4010 -> [_ w4033]
                      tunnel: w4009 -> [_ w4032]
                      tunnel: w4006 -> [_ w4031]
                      tunnel: w4005 -> [w4019 _]
                      tunnel: w4004 -> [w4015 w4029]
                      tunnel: w4003 -> [_ w4030]
                      tunnel: w4002 -> [_ w4025]
                      frame #0 {
                        n2185 = case shown="True" w4019 {
                          tunnel: w4018 -> [_ w4024]
                          tunnel: w4017 -> [_ w4023]
                          tunnel: w4016 -> [_ w4022]
                          tunnel: w4015 -> [_ w4020]
                          frame False {
                          }
                          frame True {
                            n2186 = Bundle(cluster=w4020, "amps"=w4024, "volts"=w4023, "pf"=w4022) -> (w4021:cluster{"amps":dbl, "volts":dbl, "pf":dbl})
                            n2187 = local write "ON L03-1"(w4021) -> ()
                          }
                        }
                      }
                      frame #1 {
                        n2188 = Unbundle(w4029) -> ("amps"=w4028:dbl, "volts"=w4027:dbl, "pf"=w4026:dbl)
